vi "copyToScriptRun.vi"(8 "error in (no error)":errorcluster, 10 "Path":path, 11 "ExperimentRunner in":refnum<class "ExperimentRunner.lvclass">) -> (0 "error out":errorcluster, 2 "Path out":path, 3 "ExperimentRunner out":refnum<class "ExperimentRunner.lvclass">)   [LabVIEW 2009, in "Views.lvlib" / "ExperimentControl.lvlib" / "ExperimentRunner.lvclass"]
uses:
  ExperimentRunner.lvclass
  Tools/Filing/FileSystem/FileSystem.lvclass
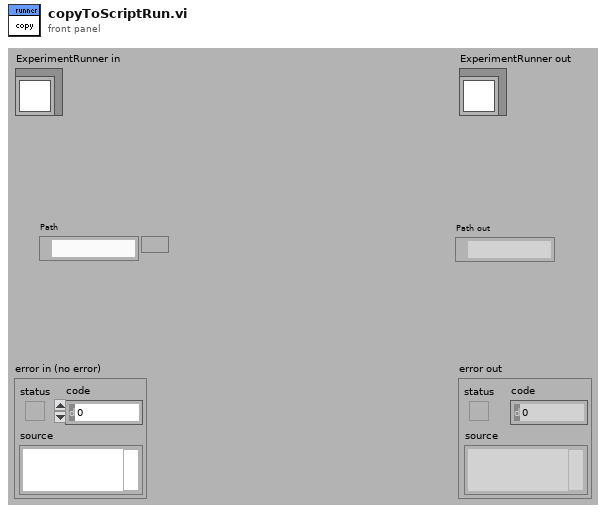
[diagram p1: front panel]
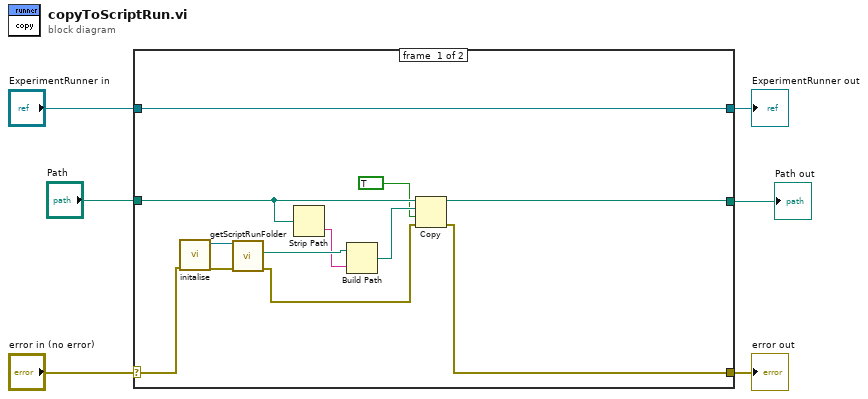
[diagram p0: block diagram]
diagram:
  n1 = case shown="No Error" "error in (no error)" {
    selector: "error in (no error)" -> [w8 w20]
    tunnel: [w12 w20] -> w5
    tunnel: [w18 w19] -> w3
    tunnel: "ExperimentRunner in" -> [w18 w19]
    tunnel: "Path" -> [w17 _]
    tunnel: [w13 _] -> w1
    frame #0 {
      n2 = call "initalise.vi"("error in (no error)"=w8) -> ("error out"=w9:errorcluster, "FileSystem out"=w10:refnum<class "FileSystem.lvclass">)  [unwired: 9 in]
      n3 = call "getScriptRunFolder.vi"("error in (no error)"=w9, "FileSystem.lvclass in"=w10) -> ("error out"=w7:errorcluster, "ScriptRunFolder"=w16:path)  [unwired: 7 in, 1 out]
      n4 = Strip Path(path=w17) -> (name=w15:string)  [unwired: 1 out]
      n5 = Build Path(base path=w16, name or relative path=w15) -> (appended path=w14:path)
      n6 = Copy(8:w7, 9:TRUE, 10:w14, 11:w17) -> (0:w12:errorcluster, 3:w13:path)  [unwired: 1 in, 1 out]
    }
    frame #1 {
    }
  }
  "error out" <- w5
  "ExperimentRunner out" <- w3
  "Path out" <- w1
